vi "WebCam.vi"() -> ()   [LabVIEW 2024]
uses:
  <vilib>/userDefined/High Color/IMAQdx.ctl
  <vilib>/vision/driver/NI_Vision_Acquisition_Software.lvlib
panel:
  out "error out":errorcluster
  in  "Record":bool
  out "Image":T1(plugin-control)
  in  "Session In":T2
  in  "stop":bool
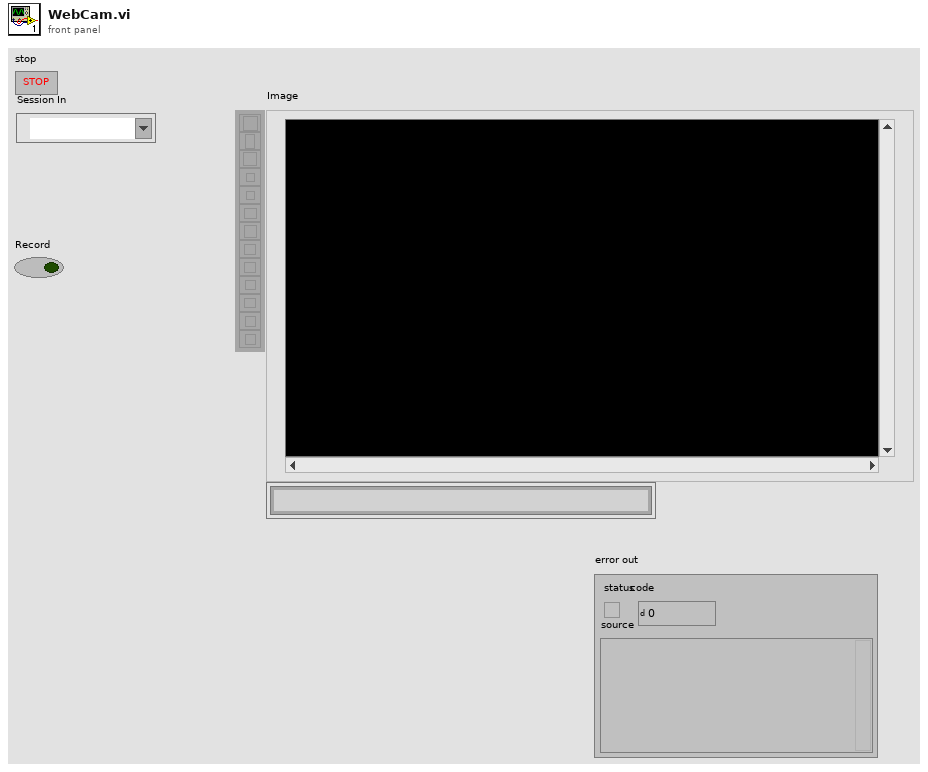
[diagram p1: front panel]
types:
  T1 = typedef "IMAQ Image.ctl" = refnum<image>
  T2 = typedef "IMAQdx.ctl" = refnum<k21>
  T3 = typedef "Image Type" = u32
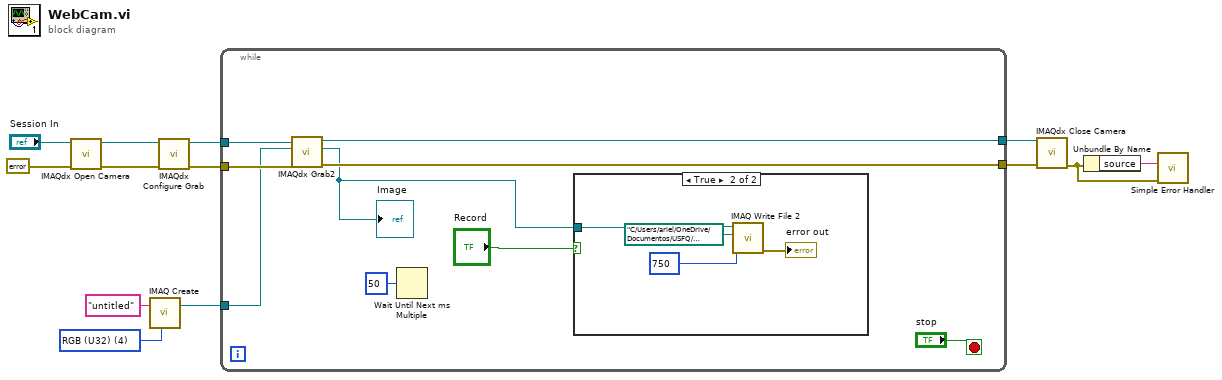
[diagram p0: block diagram]
diagram:
  w4 = T3 4 items=["Grayscale (U8)", "Grayscale (I16)", "Grayscale (SGL)", "Complex (CSG)", "RGB (U32)", "HSL (U32)", "RGB (U64)", "Grayscale (U16)"] ("Image Type")
  n1 = call <vilib>:"IMAQdx Open Camera.vi"("error in"=errorcluster {"status"=FALSE, "code"=0, "source"=""}, "Session In"="Session In") -> ("error out"=w10:errorcluster, "Session Out"=w11:T2)  [unwired: 8 in]
  n2 = call "IMAQ Create"("Image Name"="untitled", "Image Type"=w4) -> ("New Image"=w3:T1)  [unwired: 3 in, 1 out]
  n3 = call <vilib>:"IMAQdx Configure Grab.vi"("error in"=w10, "Session In"=w11) -> ("error out"=w8:errorcluster, "Session Out"=w9:T2)  [unwired: 8 in]
  n4 = while {
    tunnel: w9 -> [w21]
    tunnel: w8 -> [w20]
    tunnel: [w19] -> w7
    tunnel: [w18] -> w6
    tunnel: w3 -> [w17]
    stop <- "stop" stop-if-true
    n5 = call <vilib>:"IMAQdx Grab2.vi"("error in"=w20, "Image In"=w17, "Session In"=w21) -> ("error out"=w18:errorcluster, "Image Out"=w14:T1, "Session Out"=w19:T2)  [unwired: 5 in, 1 out]
    "Image" <- w14
    n6 = Wait Until Next ms Multiple(millisecond multiple=u32 50) -> ()  [unwired: 1 out]
    n7 = case shown="True" "Record" {
      tunnel: w14 -> [_ w26]
      frame False {
      }
      frame True {
        n8 = call-poly "IMAQ Write File 2"("Image Quality"=u32 750, "File Path"=path "C:/Users/ariel/OneDrive/Documentos/USFQ/OCTAVO SEMESTRE/EXPERIMENTAL/INTERFEROMETRIA/Recordings/test.png", "Image"=w26) -> ("error out"=→"error out":errorcluster)  [unwired: 7 in, 1 out]
      }
    }
  }
  n9 = call <vilib>:"IMAQdx Close Camera.vi"("error in"=w6, "Session In"=w7) -> ("error out"=w1:errorcluster)  [unwired: 9 in]
  n10 = Unbundle By Name(w1) -> ("source"=w2:string)
  n11 = call <vilib>:"Simple Error Handler.vi"("error source (\" \")"=w2, "error in (no error)"=w1) -> ()  [unwired: 3 in, 5 out]
